vi "AutorangeSet A0.Gains.vi"(8 "error in (no error)":errorcluster) -> (0 "error out":errorcluster)   [LabVIEW 2015]
uses:
  PXI Globals.vi
panel:
  # "Uses Multipliers Global \nand AO voltage amplitude (Vp) global\nto set\nAO Gains Global"
  # "PXI DAQ uses AO Gains Global\nto set the \nAO Gain range property node\n(allowed values 0, -20, -40  dB)"
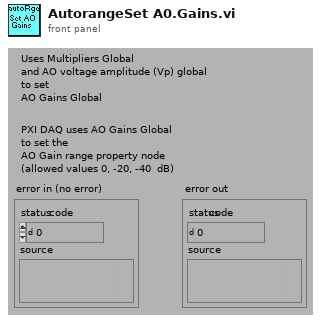
[diagram p1: front panel]
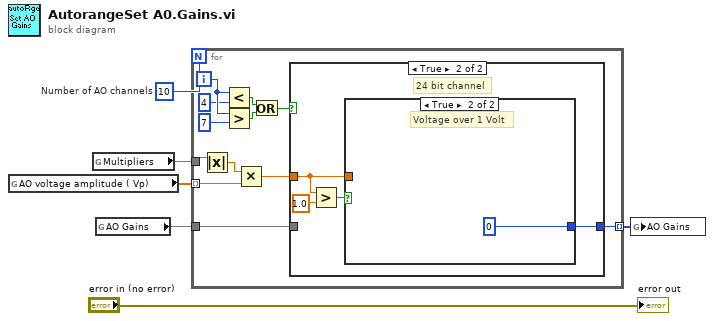
[diagram p0: block diagram]
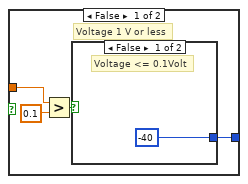
[diagram p3: hidden frame]
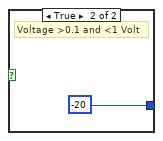
[diagram p4: hidden frame]
diagram:
  w6 = 10  # Number of AO channels
  n1 = global read "PXI Globals.vi" "AO voltage amplitude ( Vp)"() -> (w4:dbl[])
  n2 = global read "PXI Globals.vi" "Multipliers"() -> (w5)
  n3 = global read "PXI Globals.vi" "AO Gains"() -> (w3)
  n4 = for {
    N: w6 -> [_]
    tunnel: w5 -> [w18]
    tunnel: w4 -> [w17] mode=indexing
    tunnel: w3 -> [w8]
    tunnel: [w7] -> w2 mode=indexing
    i -> [w15]
    n5 = Absolute Value(x=w18) -> (abs(x)=w16:dbl)
    n6 = Less?(x=w15, y=4) -> (x < y?=w11:bool)
    n7 = Greater?(x=w15, y=7) -> (0:w12:bool)
    n8 = Multiply(x=w16, y=w17) -> (x*y=w9:dbl)
    n9 = Or(x=w11, y=w12) -> (x .or. y?=w10:bool)
    n10 = case shown="True" w10 {
      tunnel: w9 -> [_ w20]
      tunnel: w8 -> [w19 _]
      tunnel: [w19 w21] -> w7
      frame False {
        # "Not 24 bit channel"
      }
      frame True {
        # "24 bit channel"
        n11 = Greater?(x=w20, y=1.0) -> (0:w22:bool)
        n12 = case shown="True" w22 {
          tunnel: [w24 0] -> w21
          tunnel: w20 -> [w26 _]
          frame False {
            # "Voltage 1 V or less"
            n13 = Greater?(x=w26, y=0.1) -> (0:w25:bool)
            n14 = case shown="False" w25 {
              tunnel: [-40 -20] -> w24
              frame False {
                # "Voltage <= 0.1Volt"
              }
              frame True {
                # "Voltage >0.1 and <1 Volt"
              }
            }
          }
          frame True {
            # "Voltage over 1 Volt"
          }
        }
      }
    }
  }
  n15 = global write "PXI Globals.vi" "AO Gains"(w2) -> ()
  "error out" <- "error in (no error)"
